vi "SetUpAcqu.vi"() -> ()   [LabVIEW 2011]
uses:
  TDE_mode.ctl
  <vilib>/Platform/TimedLoop/XDataNode/timing_clust.ctl
  <vilib>/Platform/TimedLoop/XDataNode/nitl_modes.ctl
  <vilib>/Platform/TimedLoop/XDataNode/wakeup.ctl
  Basler - A504 Comm tool.llb/1301_BASLER_A504_TD_commands.ctl
  <vilib>/Platform/TimedLoop/XDataNode/XDataNode.xnode
  <vilib>/Platform/TimedLoop/XDataNode/XDNodeRunTimeDep.lvlib
panel:
  out "doc":picture caption="Acq mode explanation :"
  out "Period":i64
  out "Image":T1(plugin-control)
  in  "Message":string="External trig source at 3.9 kHz"
  out "FPS":u32 caption="Acq. Rate" format="%d Hz"
  out "LVF":u32 caption="Last Valid Frame"
  in  "Stop":bool
  out "error out":errorcluster
  in  "Parameters":T3={"Mode"=enum."ExSync Prog", "Frame rate"=100, "Exposure time"=160} {"Exposure time" format="%d µs"; "Frame rate" max=100000 step=1 format="%d Hz"}
  in  "Acquisition Window":T4={"Height"=128, "Left"=0, "Top"=0, "Width"=1000} {"Top" max=1022 step=2; "Left" min=0 max=1270 step=10}
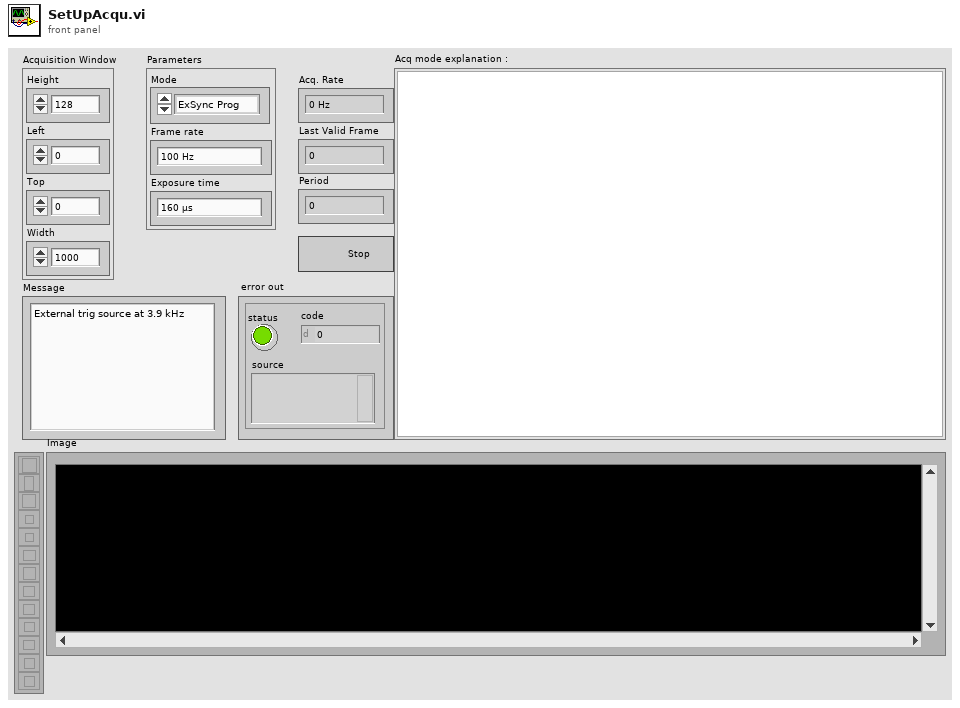
[diagram p1: front panel]
types:
  T1 = typedef "IMAQ Image.ctl" = refnum<image>
  T2 = typedef "TDE_mode.ctl" = enum16{"Free Run", "ExSync Prog", "ExSync Lev", "ExSync Edge"}
  T3 = cluster{"Mode":T2, "Frame rate":u32, "Exposure time":u32}
  T4 = cluster{"Height":u32, "Left":i32, "Top":u32, "Width":u32}
  T5 = enum8{"Enabled", "Disabled", "Disabled and Grayed Out"}
  T6 = typedef "1301_BASLER_A504_TD_commands.ctl" = enum16{"Read Status", "Exposer Time [us]", "Frame Rate", "ROI start column", "ROI width column", "ROI starting line", "ROI height in lines", "Free-Run", "ExSync programmable", "ExSync Level-controlled", "ExSync Edge-controlled", "Set Gain", "Set PosOffset", "Set NegOffset", "reset"}
  T7 = typedef "Image Type" = u32
  T8 = typedef "XDNodeRunTimeDep.lvlib/timing_clust.ctl" = cluster{"Expected End [f-1]":u64, "Actual End [f-1]":u64, "Finished Late? [f-1]":bool, "Expected End [i-1]":u64, "Actual End [i-1]":u64, "Finished Late? [i-1]":bool, "Expected Start [i]":u64, "Actual Start [i]":u64, "Expected Start [f]":u64, "Actual Start [f]":u64, "Source Name":string, "Structure Name":string, "Period":i64, "Deadline":i64, "Offset":i64, "Start":i64, "Priority":i32, "Timeout":i32, "Mode":T9, "Wakeup Reason":T10, "Error":errorcluster, "Source Type":string, "Secondary Source Type":string, "Global End Time":u64, "Global Start Time":u64, "Frame Duration":u64, "Iteration Duration":u64, "Assigned CPU":i32, "I/O Scan Engine Mode":u32}
  T9 = typedef "XDNodeRunTimeDep.lvlib/nitl_modes.ctl" = enum32{"No Change", "Process missed periods, maintain original phase", "Discard missed periods, maintain original phase", "Process missed periods, ignore original phase", "Discard missed periods, ignore original phase"}
  T10 = typedef "XDNodeRunTimeDep.lvlib/wakeup.ctl" = enum32{"Normal", "Aborted", "Asynchronous wakeup", "Timing source error", "Timed loop error", "Timeout"}
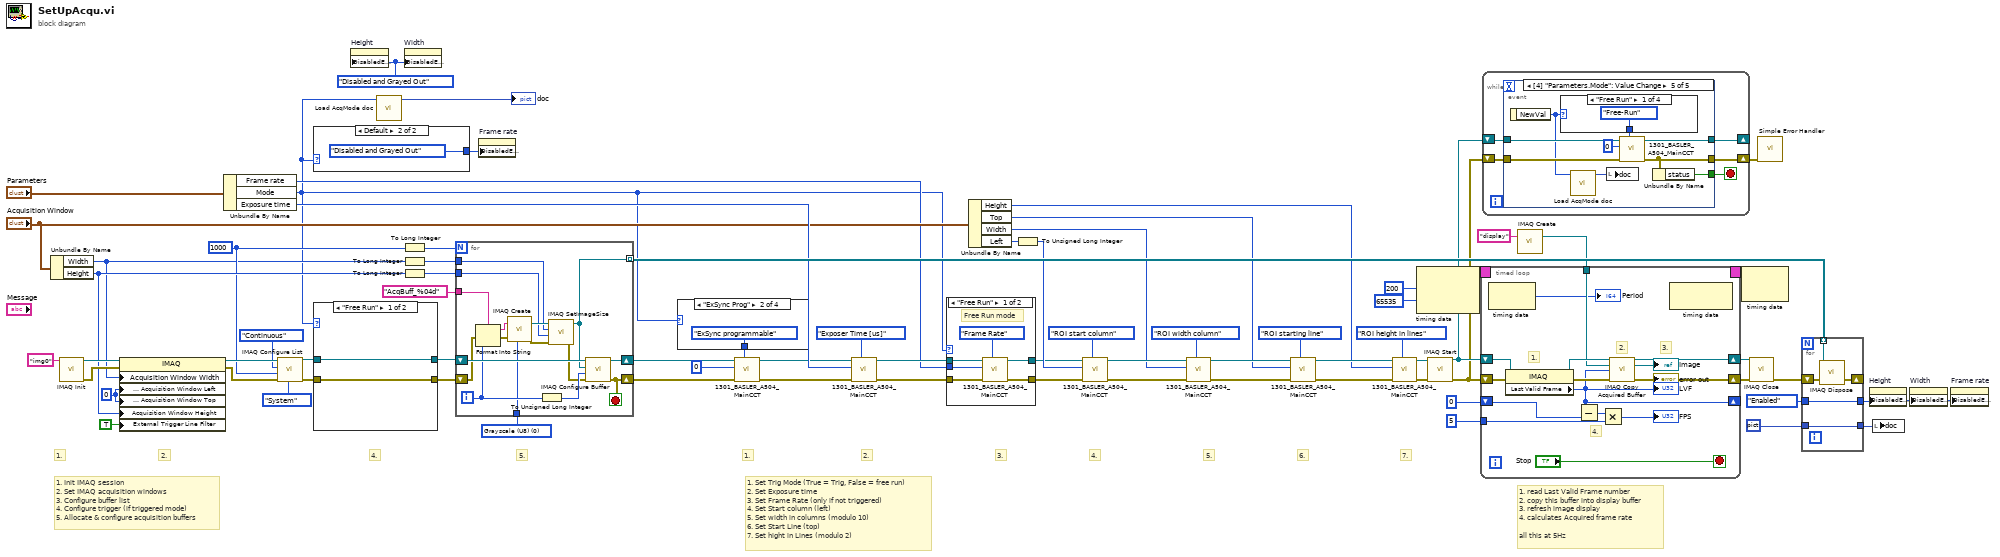
[diagram p0: block diagram]
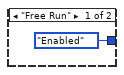
[diagram p2: hidden frame]
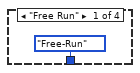
[diagram p3: hidden frame]
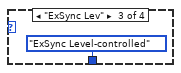
[diagram p4: hidden frame]
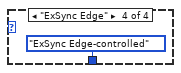
[diagram p5: hidden frame]
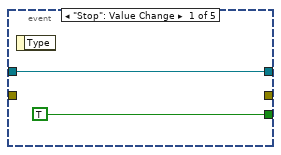
[diagram p6: hidden frame]
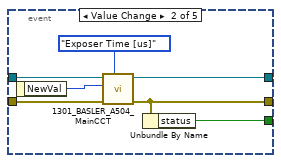
[diagram p7: hidden frame]
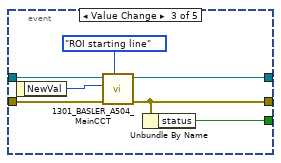
[diagram p8: hidden frame]
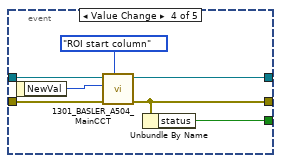
[diagram p9: hidden frame]
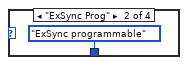
[diagram p10: hidden frame]
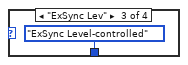
[diagram p11: hidden frame]
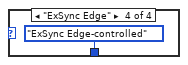
[diagram p12: hidden frame]
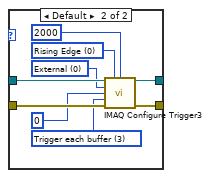
[diagram p14: hidden frame]
diagram:
  w7 = T5."Disabled and Grayed Out" ("Disabled")
  w54 = T7 0 items=["Grayscale (U8)", "Grayscale (I16)", "Grayscale (SGL)", "Complex (CSG)", "RGB (U32)", "HSL (U32)", "RGB (U64)", "Grayscale (U16)"] ("Image Type")
  w32 = u32 1000 ("Number of buffers")
  w61 = u32 0 ("Session Information : Acquisition Window Top")
  # "1. read Last Valid Frame number\n2. copy this buffer into display buffer\n3. refresh image display\n4. calculates Acquired frame rate\n\nall this at 5Hz"
  # "1."
  # "2."
  # "4."
  # "5."
  # "7."
  # "1. Init IMAQ session\n2. Set IMAQ acquisition windows\n3. Configure buffer list\n4. Configure trigger (if triggered mode)\n5. Allocate & configure acquisition buffers"
  # "1."
  # "2."
  # "3."
  # "4."
  # "5."
  # "6."
  # "1. Set Trig Mode (True = Trig, False = free run)\n2. Set Exposure time\n3. Set Frame Rate (only if not triggered)\n4. Set Start column (left)\n5. Set width in columns (modulo 10)\n6. Set Start Line (top)\n7. Set hight in Lines (modulo 2)"
  n1 = Unbundle By Name("Acquisition Window") -> ("Width"=w29:u32, "Height"=w34:u32)
  n2 = call <vilib>:"IMAQ Init.vi"("Interface Name"="img0") -> ("error out"=w53:errorcluster, "IMAQ Session Out"=w76:refnum<k11>)  [unwired: 9 in]
  n3 = property class="IMAQ"(reference=w76, error in=w53, "Acquisition Window Width"=w29, "Session Information : Acquisition Window Left"=w61, "Session Information : Acquisition Window Top"=w61, "Acquisition Window Height"=w34, "External Trigger Line Filter"=TRUE ("Acquisition Parameters : External Trigger Line Filter")) -> (reference out=w63:refnum<k11>, error out=w62:errorcluster)
  n4 = Unbundle By Name("Parameters") -> ("Frame rate"=w18:u32, "Mode"=w4:T2, "Exposure time"=w52:u32)
  n5 = call <vilib>:"IMAQ Configure List.vi"("Memory Location"=enum16{"System", "Onboard"}."System", "error in (no error)"=w62, "Number of buffers"=w32, "Continuous?"=enum16{"One-Shot", "Continuous"}."Continuous", "IMAQ Session In"=w63) -> ("error out"=w60:errorcluster, "IMAQ Session Out"=w59:refnum<k11>)  [unwired: 5 in]
  n6 = case shown="Default" w4 {
    tunnel: [T5."Enabled" ("Disabled") T5."Disabled and Grayed Out" ("Disabled")] -> w8
    frame "Free Run" {
    }
    frame Default {
    }
  }
  n7 = case shown="\"Free Run\"" w4 {
    tunnel: w60 -> [w79 w89]
    tunnel: w59 -> [w80 w88]
    tunnel: [w80 w87] -> w58
    tunnel: [w79 w86] -> w57
    frame "Free Run" {
    }
    frame Default {
      w81 = u32 3 items=["Disabled", "Trigger start of acquisition", "Trigger start of each buffer list", "Trigger each buffer", "Trigger each line (linescan)", "Trigger end of acquisition"] ("Action")
      w83 = u32 0 items=["External"=0, "RTSI"=1, "ISO In"=2, "Scaled Encoder"=5, "Software Trigger"=6] ("Type")
      w85 = u32 0 items=["Rising Edge", "Falling Edge"] ("Polarity")
      n8 = call <vilib>:"IMAQ Configure Trigger3.vi"("IMAQ Session In"=w88, "Polarity"=w85, "Frame timeout (ms)"=u32 2000, "Type"=w83, "Line Number"=u32 0, "Action"=w81, "error in (no error)"=w89) -> ("IMAQ Session Out"=w87:refnum<k11>, "error out"=w86:errorcluster)  [unwired: 2 in, 5 out]
    }
  }
  n9 = property on="Height" class="DigNum (strict)"("DisabledEnum"=w7) -> ()  [unwired: 2 in, 2 out]
  n10 = call "Load AcqMode doc.vi"("Mode"=w4) -> ("new picture"=→"doc":picture)  [unwired: 10 in]
  n11 = To Long Integer(number=w32) -> (32bit integer=w31:i32)
  n12 = To Long Integer(number=w29) -> (32bit integer=w35:i32)
  n13 = To Long Integer(number=w34) -> (32bit integer=w33:i32)
  n14 = property on="Width" class="DigNum (strict)"("DisabledEnum"=w7) -> ()  [unwired: 2 in, 2 out]
  n15 = for {
    N: w31 -> [_]
    shift-right: [w104] -> w26
    shift-left: w57 -> [w93]
    shift-right: [w102] -> w27
    shift-left: w58 -> [w103]
    tunnel: "AcqBuff_%04d" ("format string") -> [w100]
    tunnel: w54 -> [w97]
    tunnel: w35 -> [w91]
    tunnel: w33 -> [w90]
    tunnel: [w92] -> w66 mode=indexing
    i -> [w99]
    stop <- w104 stop-if-true
    n16 = Format Into String(format string=w100, error in=w93, w99) -> (resulting string=w101:string, error out=w96:errorcluster)  [unwired: 1 in]
    n17 = call "IMAQ Create"("Image Name"=w101, "Image Type"=w97, "error in (no error)"=w96) -> ("New Image"=w98:T1, "error out"=w95:errorcluster)  [unwired: 2 in]
    n18 = To Unsigned Long Integer(number=w99) -> (unsigned 32bit integer=w105:u32)
    n19 = call "IMAQ SetImageSize"("error in (no error)"=w95, "Y Resolution"=w90, "X Resolution"=w91, "Image"=w98) -> ("error out"=w94:errorcluster, "Image Out"=w92:T1)  [unwired: 1 in]
    n20 = call <vilib>:"IMAQ Configure Buffer.vi"("error in (no error)"=w94, "Buffer Number"=w105, "Image In"=w92, "IMAQ Session In"=w103) -> ("error out"=w104:errorcluster, "IMAQ Session Out"=w102:refnum<k11>)  [unwired: 6 in]
  }
  n21 = property on="Frame rate" class="DigNum (strict)"("DisabledEnum"=w8) -> ()  [unwired: 2 in, 2 out]
  n22 = case shown="\"ExSync Prog\"" w4 {
    tunnel: [1301_BASLER_A504_TD_commands."Free-Run" ("Commands") 1301_BASLER_A504_TD_commands."ExSync programmable" ("Commands") 1301_BASLER_A504_TD_commands."ExSync Level-controlled" ("Commands") 1301_BASLER_A504_TD_commands."ExSync Edge-controlled" ("Commands")] -> w51
    frame "Free Run" {
    }
    frame "ExSync Prog" {
    }
    frame "ExSync Lev" {
    }
    frame "ExSync Edge" {
    }
  }
  n23 = call "1301_BASLER_A504_MainCCT.vi"("Commands"=w51, "error in"=w26, "Parameter"=u32 0, "Session In"=w27) -> ("error out"=w25:errorcluster, "Session out"=w24:refnum<k11>)  [unwired: 5 in, 1 out]
  n24 = call "1301_BASLER_A504_MainCCT.vi"("Commands"=1301_BASLER_A504_TD_commands."Exposer Time [us]", "error in"=w25, "Parameter"=w52, "Session In"=w24) -> ("error out"=w21:errorcluster, "Session out"=w20:refnum<k11>)  [unwired: 5 in, 1 out]
  n25 = case shown="\"Free Run\"" w4 {
    tunnel: w21 -> [w114 w116]
    tunnel: w20 -> [w113 w117]
    tunnel: [w112 w117] -> w19
    tunnel: w18 -> [w111 _]
    tunnel: [w110 w116] -> w17
    frame "Free Run" {
      # "Free Run mode"
      n26 = call "1301_BASLER_A504_MainCCT.vi"("Commands"=1301_BASLER_A504_TD_commands."Frame Rate", "error in"=w114, "Parameter"=w111, "Session In"=w113) -> ("error out"=w110:errorcluster, "Session out"=w112:refnum<k11>)  [unwired: 5 in, 1 out]
    }
    frame Default {
      # "TRIG mode"
    }
  }
  n27 = Unbundle By Name("Acquisition Window") -> ("Height"=w36:u32, "Top"=w37:u32, "Width"=w38:u32, "Left"=w39:i32)
  n28 = To Unsigned Long Integer(number=w39) -> (unsigned 32bit integer=w30:u32)
  n29 = call "1301_BASLER_A504_MainCCT.vi"("Commands"=1301_BASLER_A504_TD_commands."ROI start column", "error in"=w17, "Parameter"=w30, "Session In"=w19) -> ("error out"=w44:errorcluster, "Session out"=w41:refnum<k11>)  [unwired: 5 in, 1 out]
  n30 = call "1301_BASLER_A504_MainCCT.vi"("Commands"=1301_BASLER_A504_TD_commands."ROI width column", "error in"=w44, "Parameter"=w38, "Session In"=w41) -> ("error out"=w45:errorcluster, "Session out"=w42:refnum<k11>)  [unwired: 5 in, 1 out]
  n31 = call "1301_BASLER_A504_MainCCT.vi"("Commands"=1301_BASLER_A504_TD_commands."ROI starting line", "error in"=w45, "Parameter"=w37, "Session In"=w42) -> ("error out"=w46:errorcluster, "Session out"=w43:refnum<k11>)  [unwired: 5 in, 1 out]
  n32 = call "1301_BASLER_A504_MainCCT.vi"("Commands"=1301_BASLER_A504_TD_commands."ROI height in lines", "error in"=w46, "Parameter"=w36, "Session In"=w43) -> ("error out"=w22:errorcluster, "Session out"=w23:refnum<k11>)  [unwired: 5 in, 1 out]
  n33 = node-c288(i64 200 ("Period"), 65535 ("Priority")) -> (w73:T8)
  n34 = call <vilib>:"IMAQ Start.vi"("error in (no error)"=w22, "IMAQ Session In"=w23) -> ("error out"=w10:errorcluster, "IMAQ Session Out"=w12:refnum<k11>)  [unwired: 8 in]
  n35 = while {
    shift-right: [w120] -> _
    shift-left: w12 -> [w121]
    shift-right: [w119] -> w11
    shift-left: w10 -> [w118]
    stop <- w122 stop-if-true
    n36 = event shown="[4] \"Parameters.Mode\": Value Change" {
      selector: _ -> [_ _ _ _ _]
      dyn-events: _ -> [_ _ _ _ _]
      timeout: _ -> [_ _ _ _ _]
      tunnel: [TRUE w127 w134 w141 w151] -> w122
      tunnel: w121 -> [w123 w130 w137 w144 w153]
      tunnel: [w123 w129 w136 w143 w152] -> w120
      tunnel: [_ w126 w133 w140 w150] -> w119
      tunnel: w118 -> [_ w125 w132 w139 w149]
      event "Stop": Value Change {
        n37 = event-data() -> ()  [unwired: 1 in, 1 out]
      }
      event "Parameters.Exposure time": Value Change {
        n38 = event-data() -> ("NewVal"=w128:u32)  [unwired: 1 in]
        n39 = call "1301_BASLER_A504_MainCCT.vi"("Commands"=1301_BASLER_A504_TD_commands."Exposer Time [us]", "error in"=w125, "Parameter"=w128, "Session In"=w130) -> ("error out"=w126:errorcluster, "Session out"=w129:refnum<k11>)  [unwired: 5 in, 1 out]
        n40 = Unbundle By Name(w126) -> ("status"=w127:bool)
      }
      event "Acquisition Window.Top": Value Change {
        n41 = event-data() -> ("NewVal"=w135:u32)  [unwired: 1 in]
        n42 = call "1301_BASLER_A504_MainCCT.vi"("Commands"=1301_BASLER_A504_TD_commands."ROI starting line", "error in"=w132, "Parameter"=w135, "Session In"=w137) -> ("error out"=w133:errorcluster, "Session out"=w136:refnum<k11>)  [unwired: 5 in, 1 out]
        n43 = Unbundle By Name(w133) -> ("status"=w134:bool)
      }
      event "Acquisition Window.Left": Value Change {
        n44 = event-data() -> ("NewVal"=w142:i32)  [unwired: 1 in]
        n45 = call "1301_BASLER_A504_MainCCT.vi"("Commands"=1301_BASLER_A504_TD_commands."ROI start column", "error in"=w139, "Parameter"=w142, "Session In"=w144) -> ("error out"=w140:errorcluster, "Session out"=w143:refnum<k11>)  [unwired: 5 in, 1 out]
        n46 = Unbundle By Name(w140) -> ("status"=w141:bool)
      }
      event Value Change {
        n47 = event-data() -> ("NewVal"=w146:T2)  [unwired: 1 in]
        n48 = case shown="\"Free Run\"" w146 {
          tunnel: [1301_BASLER_A504_TD_commands."Free-Run" ("Commands") 1301_BASLER_A504_TD_commands."ExSync programmable" ("Commands") 1301_BASLER_A504_TD_commands."ExSync Level-controlled" ("Commands") 1301_BASLER_A504_TD_commands."ExSync Edge-controlled" ("Commands")] -> w154
          frame "Free Run" {
          }
          frame "ExSync Prog" {
          }
          frame "ExSync Lev" {
          }
          frame "ExSync Edge" {
          }
        }
        n49 = call "Load AcqMode doc.vi"("Mode"=w146) -> ("new picture"=w147:picture)  [unwired: 10 in]
        n50 = local write "doc"(w147) -> ()
        n51 = call "1301_BASLER_A504_MainCCT.vi"("Commands"=w154, "error in"=w149, "Parameter"=u32 0, "Session In"=w153) -> ("error out"=w150:errorcluster, "Session out"=w152:refnum<k11>)  [unwired: 5 in, 1 out]
        n52 = Unbundle By Name(w150) -> ("status"=w151:bool)
      }
    }
  }
  n53 = call "IMAQ Create"("Image Name"="display") -> ("New Image"=w13:T1)  [unwired: 4 in, 1 out]
  n54 = timed-loop {
    timing: w73 -> [_]
    timing-out: [_] -> w72
    shift-right: [w166] -> w71
    shift-left: w10 -> [w168]
    shift-right: [w164] -> w70
    shift-left: w12 -> [w173]
    shift-right: [w161] -> _
    shift-left: u32 0 ("Last Valid Frame") -> [w172]
    tunnel: u32 5 ("y") -> [w169]
    tunnel: w13 -> [w162]
    stop <- "Stop" stop-if-true
    # "4."
    # "3."
    # "2."
    # "1."
    n55 = node-c288() -> (→"Period":i64)  [unwired: 1 in]
    n56 = property class="IMAQ"(reference=w173, error in=w168) -> (reference out=w165:refnum<k11>, error out=w167:errorcluster, "Last Valid Frame"=w161:u32)
    "LVF" <- w161
    n57 = Subtract(x=w161, y=w172) -> (x-y=w171:u32)
    n58 = Multiply(x=w171, y=w169) -> (x*y=→"FPS":u32)
    n59 = call <vilib>:"IMAQ Copy Acquired Buffer.vi"("IMAQ Session In"=w165, "Image In"=w162, "Buffer Number"=w161, "error in (no error)"=w167) -> ("IMAQ Session Out"=w164:refnum<k11>, "Image Out"=→"Image":T1, "error out"=w166:errorcluster)  [unwired: 7 in, 2 out]
    "error out" <- w166
    n60 = node-c288() -> ()  [unwired: 1 in, 1 out]
  }
  n61 = node-c288(w72) -> ()  [unwired: 1 out]
  n62 = call <vilib>:"IMAQ Close.vi"("error in (no error)"=w71, "IMAQ Session In"=w70) -> ("error out"=w67:errorcluster)  [unwired: 9 in]
  n63 = call <vilib>:"Simple Error Handler.vi"("error in (no error)"=w11) -> ()  [unwired: 4 in, 5 out]
  n64 = for {
    tunnel: w66 -> [w180] mode=indexing
    shift-right: [w179] -> _
    shift-left: w67 -> [w181]
    tunnel: [w178] -> w6
    tunnel: T5."Enabled" ("Disabled") -> [w178]
    tunnel: [w177] -> w2
    tunnel: picture data[5B] ("picture") -> [w177]
    n65 = call "IMAQ Dispose"("Image"=w180, "error in (no error)"=w181) -> ("error out"=w179:errorcluster)  [unwired: 4 in]
  }
  n66 = property on="Height" class="DigNum (strict)"("DisabledEnum"=w6) -> ()  [unwired: 2 in, 2 out]
  n67 = local write "doc"(w2) -> ()
  n68 = property on="Width" class="DigNum (strict)"("DisabledEnum"=w6) -> ()  [unwired: 2 in, 2 out]
  n69 = property on="Frame rate" class="DigNum (strict)"("DisabledEnum"=w6) -> ()  [unwired: 2 in, 2 out]
